vi "openini.vi"(0 "INI file name":string="cs130.ini") -> (1 "refnum":refnum<k1>, 2 "appended path":path)   [LabVIEW 2017]
doc: "Utility VI to generate path for the configuration file (INI) to current directory\nHandles the LabView bug which generates a bad path at runtime."
uses:
  <vilib>/Utility/config.llb/NI_LVConfig.lvlib
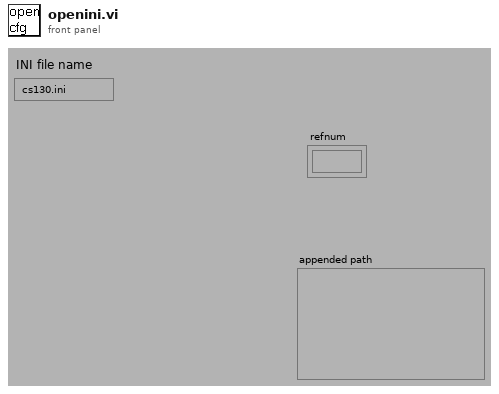
[diagram p1: front panel]
types:
  T1 = typedef "NI_LVConfig.lvlib/Config Data RefNum.ctl" = refnum<k1>
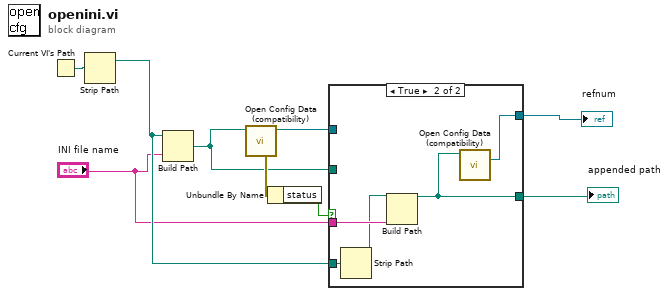
[diagram p0: block diagram]
diagram:
  n1 = Current VI's Path() -> (path=w9:path)
  n2 = Strip Path(path=w9) -> (stripped path=w5:path)  [unwired: 1 out]
  n3 = Build Path(base path=w5, name or relative path="INI file name") -> (appended path=w2:path)
  n4 = call <vilib>:"Open Config Data (compatibility).vi"("configuration file path"=w2) -> ("error out"=w8:errorcluster, "refnum"=w6:T1)  [unwired: 8 in, 1 out]
  n5 = Unbundle By Name(w8) -> ("status"=w7:bool)
  n6 = case shown="True" w7 {
    tunnel: w6 -> [w11 _]
    tunnel: [w11 w13] -> w1
    tunnel: w5 -> [_ w16]
    tunnel: "INI file name" -> [_ w15]
    tunnel: [w10 w12] -> w3
    tunnel: w2 -> [w10 _]
    frame False {
    }
    frame True {
      n7 = Strip Path(path=w16) -> (stripped path=w14:path)  [unwired: 1 out]
      n8 = Build Path(base path=w14, name or relative path=w15) -> (appended path=w12:path)
      n9 = call <vilib>:"Open Config Data (compatibility).vi"("configuration file path"=w12) -> ("refnum"=w13:T1)  [unwired: 8 in, 2 out]
    }
  }
  "appended path" <- w3
  "refnum" <- w1
